vi "strip formatting.vi"(1 "result string 2":string) -> (0 "result string":string)   [LabVIEW 2018]
uses:
  <vilib>/regexp/Match Regular Expression.xnode
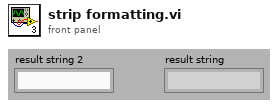
[diagram p1: front panel]
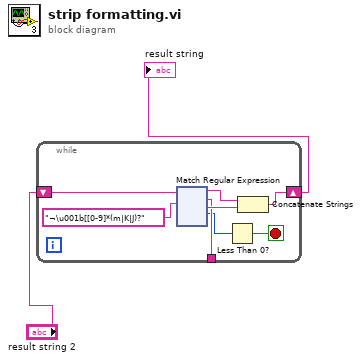
[diagram p0: block diagram]
diagram:
  n1 = while {
    shift-right: [w7] -> w2
    shift-left: "result string 2" -> [w4]
    tunnel: [w6] -> _
    stop <- w5 stop-if-true
    n2 = xnode "Match Regular Expression"("input string"=w4, "regular expression"="¬\u001b[[0-9]*(m|K|J)?" ("search string")) -> ("before match"=w8:string, "whole match"=w6:string, "after match"=w9:string, "offset past match"=w3:i32)  [unwired: 4 in, 1 out]
    n3 = Less Than 0?(x=w3) -> (x < 0?=w5:bool)
    n4 = Concatenate Strings(w8, w9) -> (w7:string)
  }
  "result string" <- w2
